vi "ConvertActions.vi"(11 "Actions":T1(array[cluster])) -> (3 "ActionString":string)   [LabVIEW 2021, in "ButtonBarFlow.lvlib"]
uses:
  ButtonBarFlow.lvlib
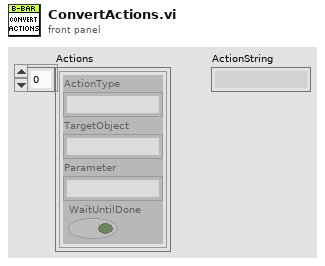
[diagram p1: front panel]
types:
  T1 = cluster{"ActionType":string, "TargetObject":string, "Parameter":string, "WaitUntilDone":bool}[]
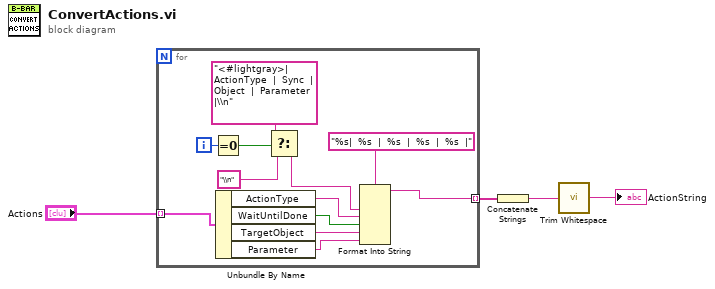
[diagram p0: block diagram]
diagram:
  n1 = for {
    tunnel: "Actions" -> [w16] mode=indexing
    tunnel: [w11] -> w3 mode=indexing
    i -> [w10]
    n2 = Equal To 0?(x=w10) -> (x = 0?=w6:bool)
    n3 = Unbundle By Name(w16) -> ("ActionType"=w15:string, "WaitUntilDone"=w5:bool, "TargetObject"=w14:string, "Parameter"=w13:string)
    n4 = Select(t="<#lightgray>|  ActionType  |  Sync  |  Object  |  Parameter  |\\n", s=w6, f="\\n") -> (s? t:f=w7:string)
    n5 = Format Into String(format string="%s|  %s  |  %s  |  %s  |  %s  |", w7, w15, w5, w14, w13) -> (resulting string=w11:string)  [unwired: 2 in, 1 out]
  }
  n6 = Concatenate Strings(w3) -> (w4:string)
  n7 = call <vilib>:"Trim Whitespace.vi"("string"=w4) -> ("trimmed string"=→"ActionString":string)  [unwired: 1 in]
